vi "WSVCAP SHL FPGA LL I2C FIFO Manager - Pre and Post.vi"(0 "64 Bit Data In":u64, 7 "timeout in ms (-1)":i32, 11 "error in (no error)":errorcluster, 13 "Operation":T1) -> (8 "Timed Out":bool, 10 "64 Bit Data Out":u64, 15 "error out":errorcluster)   [LabVIEW 2017]
uses:
  Type Defs/WSVCAP SHL FIFO Operation Enum.ctl
  <vilib>/rvi/DataTransferAndStorage/Container/XNode/niFpgaContainer.xnode
  <vilib>/rvi/FIFO/Fifo_Resource/nirvififoEmulationWrite.vi
  <vilib>/rvi/FIFO/Fifo_Resource/nirvififoEmulationRead.vi
panel:
  out "elements":u64[](array[numeric]) format="%.0x"
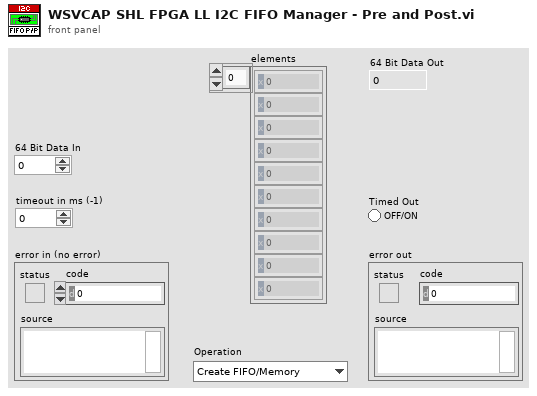
[diagram p1: front panel]
types:
  T1 = typedef "WSVCAP SHL FIFO Operation Enum.ctl" = enum16{"Create FIFO/Memory", "Get Write FIFO Status", "Get Read FIFO Status", "Put Element in Write", "Put Element in Read", "Get Element from Write", "Get Element from Read"}
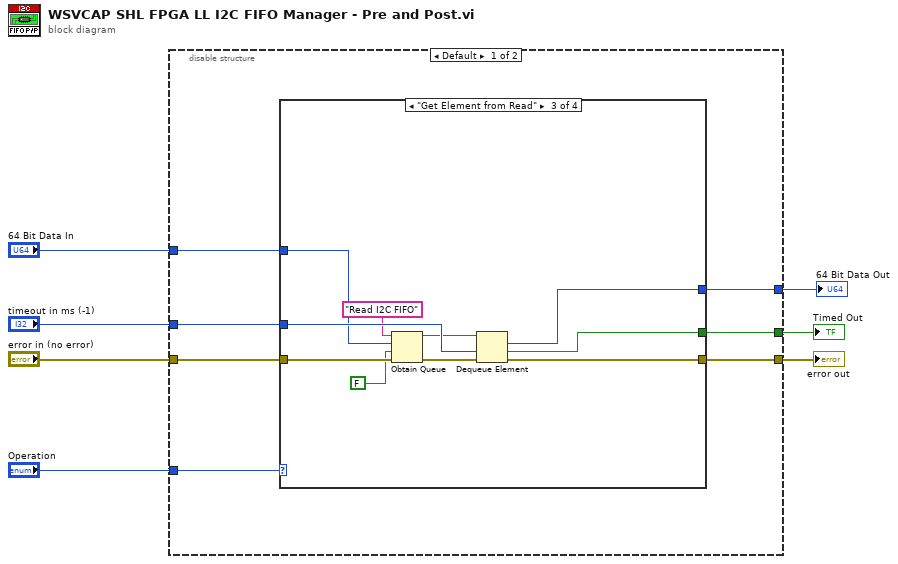
[diagram p0: block diagram]
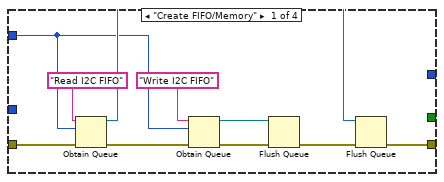
[diagram p2: hidden frame]
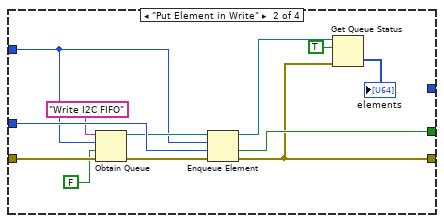
[diagram p3: hidden frame]
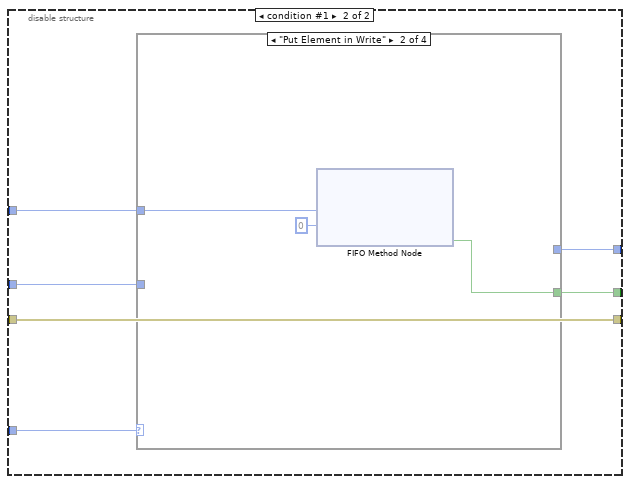
[diagram p5: hidden frame]
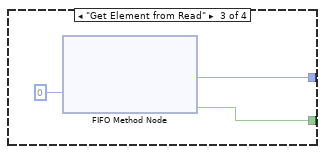
[diagram p7: hidden frame]
diagram:
  n1 = disable-structure shown="Default" {
    disable-tunnel: "Operation" -> [w14 w53]
    disable-tunnel: "error in (no error)" -> [w13 w48]
    disable-tunnel: [w12 w48] -> w5
    disable-tunnel: "64 Bit Data In" -> [w11 w52]
    disable-tunnel: "timeout in ms (-1)" -> [w10 w51]
    disable-tunnel: [w9 w50] -> w2
    disable-tunnel: [w8 w49] -> w1
    frame condition #0 (active) {
      n2 = case shown="\"Get Element from Read\"" w14 {
        tunnel: [w18 w26 w45 w47] -> w12
        tunnel: w13 -> [w22 w34 w43 w47]
        tunnel: w11 -> [w15 w30 w37 _]
        tunnel: w10 -> [_ w36 w46 _]
        tunnel: [_ w35 w44 _] -> w9
        tunnel: [_ _ w38 _] -> w8
        frame "Create FIFO/Memory" {
          n3 = Obtain Queue(name (unnamed)="Read I2C FIFO", element data type=w15, error in (no error)=w22) -> (queue out=w17:refnum<queue>, error out=w21:errorcluster)  [unwired: 2 in, 1 out]
          n4 = Obtain Queue(name (unnamed)="Write I2C FIFO", element data type=w15, error in (no error)=w21) -> (queue out=w16:refnum<queue>, error out=w20:errorcluster)  [unwired: 2 in, 1 out]
          n5 = Flush Queue(queue=w16, error in (no error)=w20) -> (error out=w19:errorcluster)  [unwired: 2 out]
          n6 = Flush Queue(queue=w17, error in (no error)=w19) -> (error out=w18:errorcluster)  [unwired: 2 out]
        }
        frame "Put Element in Write" {
          n7 = Obtain Queue(name (unnamed)="Write I2C FIFO", element data type=w30, create if not found? (T)=FALSE, error in (no error)=w34) -> (queue out=w31:refnum<queue>, error out=w33:errorcluster)  [unwired: 1 in, 1 out]
          n8 = Enqueue Element(queue=w31, element=w30, timeout in ms (-1)=w36, error in (no error)=w33) -> (queue out=w27:refnum<queue>, timed out?=w35:bool, error out=w26:errorcluster)
          n9 = Get Queue Status(queue=w27, return elements? (F)=TRUE, error in (no error)=w26) -> (elements=→"elements":u64[])  [unwired: 7 out]
        }
        frame "Get Element from Read" {
          n10 = Obtain Queue(name (unnamed)="Read I2C FIFO", element data type=w37, create if not found? (T)=FALSE, error in (no error)=w43) -> (queue out=w40:refnum<queue>, error out=w42:errorcluster)  [unwired: 1 in, 1 out]
          n11 = Dequeue Element(queue=w40, timeout in ms (-1)=w46, error in (no error)=w42) -> (element=w38:u64, timed out?=w44:bool, error out=w45:errorcluster)  [unwired: 1 out]
        }
        frame Default {
        }
      }
    }
    frame condition #1 {
      n12 = case shown="\"Put Element in Write\"" w53 {
        tunnel: w52 -> [_ w55 _ _]
        tunnel: w51 -> [_ _ _ _]
        tunnel: [_ w56 w58 _] -> w50
        tunnel: [_ _ w59 _] -> w49
        frame "Create FIFO/Memory" {
        }
        frame "Put Element in Write" {
          n13 = xnode ("FIFO Method Node")("Element"=w55, "Timeout"=0) -> ("Timed Out?"=w56:bool)  [unwired: 1 in, 1 out]
        }
        frame "Get Element from Read" {
          n14 = xnode ("FIFO Method Node")("Timeout"=0) -> ("Element"=w59:u64, "Timed Out?"=w58:bool)  [unwired: 1 in, 1 out]
        }
        frame Default {
        }
      }
    }
  }
  "error out" <- w5
  "Timed Out" <- w2
  "64 Bit Data Out" <- w1
